vi "BoxMoy20.vi"(10 "all rows":dbl[](array[numeric]), 11 "Numérique":dbl) -> (3 "Tableau 2":dbl[](array[numeric]))   [LabVIEW 2023]
uses:
  <vilib>/Analysis/baseanly.llb/Mean (DBL).vi
  <vilib>/Analysis/NI_AALBase.lvlib
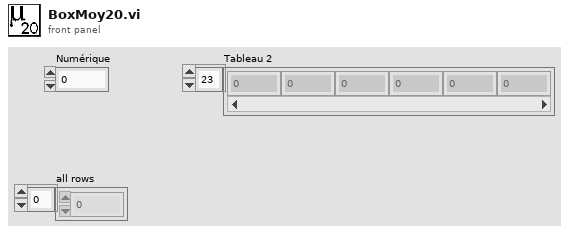
[diagram p1: front panel]
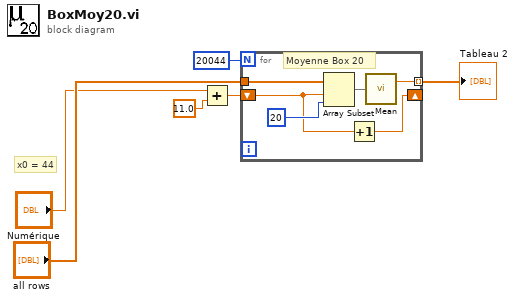
[diagram p0: block diagram]
diagram:
  # "x0 = 44"
  n1 = Add(x="Numérique", y=11.0) -> (x+y=w3:dbl)
  n2 = for {
    N: 20044 -> [_]
    shift-right: [w11] -> _
    shift-left: w3 -> [w10]
    tunnel: [w9] -> w6 mode=indexing
    tunnel: "all rows" -> [w8]
    # "Moyenne Box 20"
    n3 = Array Subset(array=w8, index=w10, length=20 ("longueur")) -> (w7:dbl[])
    n4 = Increment(x=w10) -> (x+1=w11:dbl)
    n5 = call-poly <vilib>:"Mean.vi"("X"=w7) -> ("mean"=w9:dbl)  [unwired: 1 out]
  }
  "Tableau 2" <- w6
